vi "RefreshUI Event.vi"(7 "Refresh (T)":bool=TRUE, 8 "error in (no error)":errorcluster, 11 "References in":T1) -> (0 "error out":errorcluster, 3 "References out":T1)   [LabVIEW 2013, in "Shared Memory editor node.lvclass"]
doc: "This VI triggers a refresh event in the UI and the table."
uses:
  Shared Memory editor node.lvclass
  <vilib>/NI/DCAF/Tag Editor Core/Table API/Table Manager/references.ctl
  <vilib>/NI/Configuration Framework/Node/StopEvent.ctl
  <vilib>/NI/Configuration Framework/Node/RefreshUIEvent.ctl
  <vilib>/NI/Configuration Framework/Node/CacheState.ctl
  <vilib>/NI/Configuration Framework/Node/NodeChangeEvent.ctl
  <vilib>/NI/Configuration Framework/Node/NodeRef.ctl
  <vilib>/NI/Configuration Framework/Node/NISE_CEF_Node.lvclass
  <vilib>/NI/DCAF/Tag Editor Core/Table API/Available Tag Menu/channel action event.ctl
  <vilib>/NI/DCAF/Tag Editor Core/Table API/Available Tag Menu/dialog output action.ctl
  <vilib>/NI/Tag Bus Module Framework/channel/TBM channel.lvclass
  <vilib>/NI/Tag Bus/tag/tag descriptor.lvclass
  <vilib>/NI/DCAF/Tag Editor Core/Table API/Table Manager/Call Back Ref Type Def.ctl
  <vilib>/NI/DCAF/Tag Editor Core/Configuration Editor/Classes/Engine Parent/Engine Parent Editor Node.lvclass
  <vilib>/NI/DCAF/Tag Editor Core/Configuration Editor/Classes/Module editor node/module editor node.lvclass
  <vilib>/NI/AMC/Message Queue.ctl
  <vilib>/NI/AMC/Message.ctl
  <vilib>/NI/Tools/Keyed Array/KeyedArray.ctl
  <vilib>/NI/Configuration Framework/Node/UserEventRef.ctl
  <vilib>/NI/Configuration Framework/Controls/EventCluster.ctl
  <vilib>/NI/DCAF/Tag Editor Core/Table API/Table Manager.lvlib
  <vilib>/NI/Tools/Keyed Array/Tools_KeyedArray.lvlib
  <vilib>/NI/AMC/AMC.lvlib
  <vilib>/NI/Configuration Framework/NISE_CEF_TreeControl.lvlib
  <vilib>/NI/DCAF/Tag Editor Core/Table API/Table Manager/Table Manager.lvclass
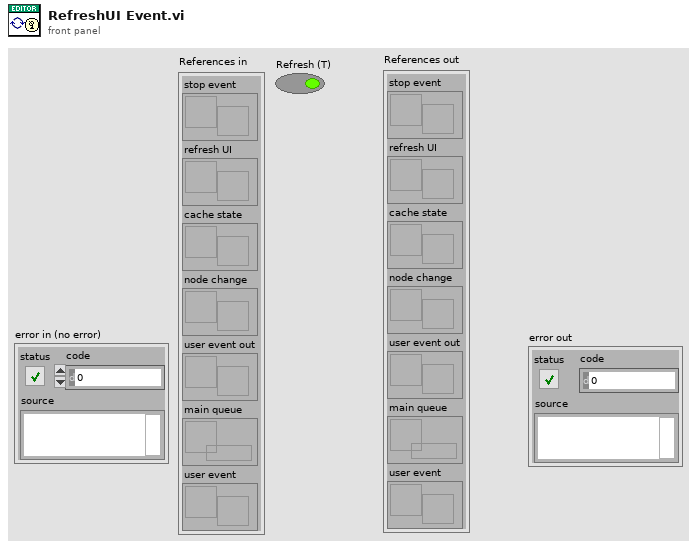
[diagram p1: front panel]
types:
  T1 = typedef "Table Manager.lvlib/Table Manager.lvclass/references.ctl" = cluster{"stop event":T2, "refresh UI":T3, "cache state":T4, "node change":T5, "user event out":refnum<user-event>, "main queue":T6, "user event":T7}
  T2 = typedef "NISE_CEF_Node.lvclass/StopEvent.ctl" = refnum<user-event>
  T3 = typedef "NISE_CEF_Node.lvclass/RefreshUIEvent.ctl" = refnum<user-event>
  T4 = typedef "NISE_CEF_Node.lvclass/CacheState.ctl" = refnum<user-event>
  T5 = typedef "NISE_CEF_Node.lvclass/NodeChangeEvent.ctl" = refnum<user-event>
  T6 = typedef "AMC.lvlib/Message Queue.ctl" = refnum<queue>
  T7 = typedef "NISE_CEF_Node.lvclass/UserEventRef.ctl" = refnum<user-event>
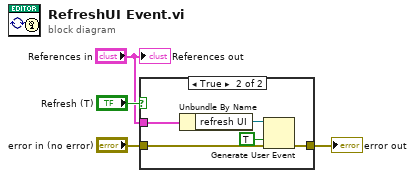
[diagram p0: block diagram]
diagram:
  n1 = case shown="True" "Refresh (T)" {
    tunnel: "error in (no error)" -> [w5 w9]
    tunnel: [w5 w8] -> w2
    tunnel: "References in" -> [_ w7]
    frame False {
    }
    frame True {
      n2 = Unbundle By Name(w7) -> ("refresh UI"=w10:T3)
      n3 = Generate User Event(user event=w10, event data cluster=TRUE ("event data"), error in=w9) -> (error out=w8:errorcluster)  [unwired: 1 in, 1 out]
    }
  }
  "error out" <- w2
  "References out" <- "References in"
